vi "FeedbackDecode_VariablesToString_Array.vi"(3 "Format":string="%0.2f", 4 "Terminate?":bool=TRUE, 5 "ValueIn":dbl[](array[numeric]), 6 "FieldName":string, 7 "Type":enum16{"Normal", "Matlab"}(ring)=enum."Matlab") -> (1 "StringOut":string)   [LabVIEW 2020]
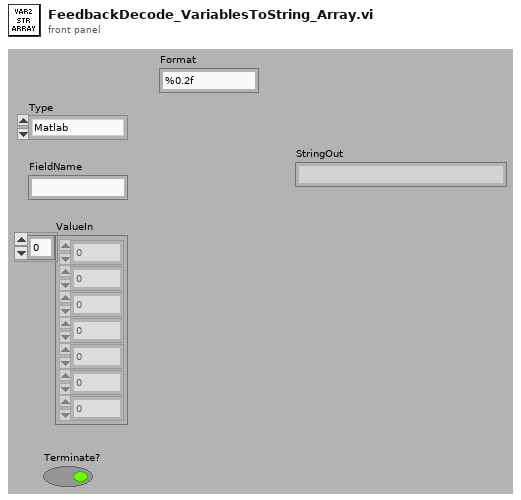
[diagram p1: front panel]
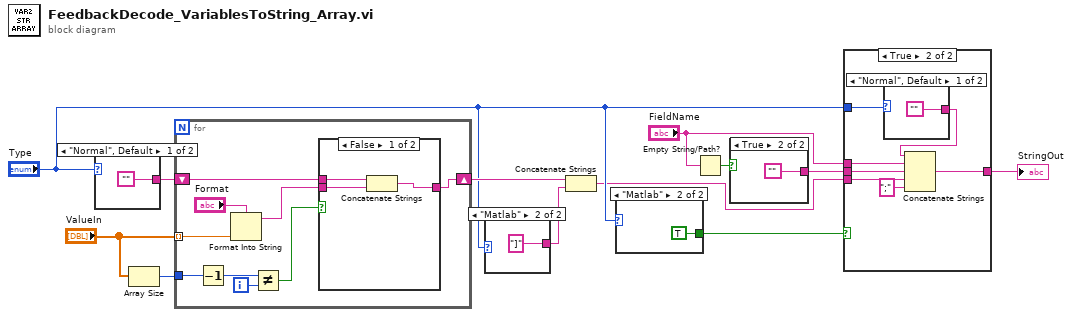
[diagram p0: block diagram]
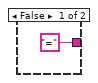
[diagram p2: hidden frame]
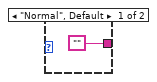
[diagram p3: hidden frame]
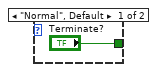
[diagram p4: hidden frame]
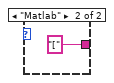
[diagram p5: hidden frame]
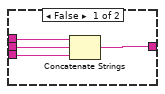
[diagram p6: hidden frame]
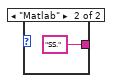
[diagram p7: hidden frame]
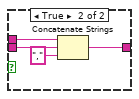
[diagram p8: hidden frame]
diagram:
  n1 = case shown="\"Normal\", Default" "Type" {
    tunnel: ["" "["] -> w10
    frame "Normal", Default {
    }
    frame "Matlab" {
    }
  }
  n2 = Array Size(array="ValueIn") -> (size(s)=w12:i32)
  n3 = for {
    tunnel: "ValueIn" -> [w23] mode=indexing
    shift-right: [w22] -> w6
    shift-left: w10 -> [w21]
    tunnel: w12 -> [w19]
    i -> [w17]
    n4 = Decrement(x=w19) -> (x-1=w18:i32)
    n5 = Format Into String(format string="Format", w23) -> (resulting string=w20:string)  [unwired: 2 in, 1 out]
    n6 = Not Equal?(x=w18, y=w17) -> (x != y?=w16:bool)
    n7 = case shown="False" w16 {
      tunnel: [w24 w30] -> w22
      tunnel: w21 -> [w26 w29]
      tunnel: w20 -> [w25 w28]
      frame False {
        n8 = Concatenate Strings(w26, w25) -> (w24:string)
      }
      frame True {
        n9 = Concatenate Strings(w29, w28, "," ("string")) -> (w30:string)
      }
    }
  }
  n10 = case shown="\"Matlab\"" "Type" {
    tunnel: ["" "]"] -> w5
    frame "Normal", Default {
    }
    frame "Matlab" {
    }
  }
  n11 = Concatenate Strings(w6, w5) -> (w3:string)
  n12 = case shown="\"Matlab\"" "Type" {
    tunnel: ["Terminate?" TRUE ("Terminate?")] -> w7
    frame "Normal", Default {
    }
    frame "Matlab" {
    }
  }
  n13 = Empty String/Path?(string/path="FieldName") -> (empty?=w1:bool)
  n14 = case shown="True" w1 {
    tunnel: ["=" ("string") ""] -> w9
    frame False {
    }
    frame True {
    }
  }
  n15 = case shown="True" w7 {
    tunnel: "FieldName" -> [w40 w47]
    tunnel: w9 -> [w39 w46]
    tunnel: w3 -> [w38 w45]
    tunnel: [w37 w43] -> w8
    tunnel: "Type" -> [_ w41]
    frame False {
      n16 = Concatenate Strings(w40, w39, w38) -> (w37:string)
    }
    frame True {
      n17 = case shown="\"Normal\", Default" w41 {
        tunnel: ["" "SS."] -> w42
        frame "Normal", Default {
        }
        frame "Matlab" {
        }
      }
      n18 = Concatenate Strings(w42, w47, w46, w45, ";" ("string")) -> (w43:string)
    }
  }
  "StringOut" <- w8
